vi "Cauchy PDF.vi"(9 "b":dbl=1.0, 10 "a":dbl, 11 "x":dbl) -> (0 "error":i32, 3 "pdf(x)":dbl=0.3183098861837907)   [LabVIEW 2014, in "NI_Gmath.lvlib"]
doc: "Computes the continuous probability density function (PDF) of various distributions. You must manually select the polymorphic instance to use."
uses:
  NI_Gmath.lvlib
  st_error_code.ctl
panel:
  # "Cauchy PDF"
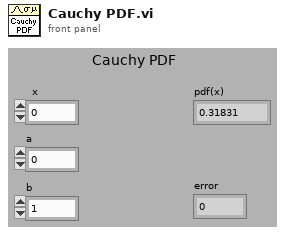
[diagram p1: front panel]
types:
  T1 = typedef "NI_Gmath.lvlib/st_error_code.ctl" = i32
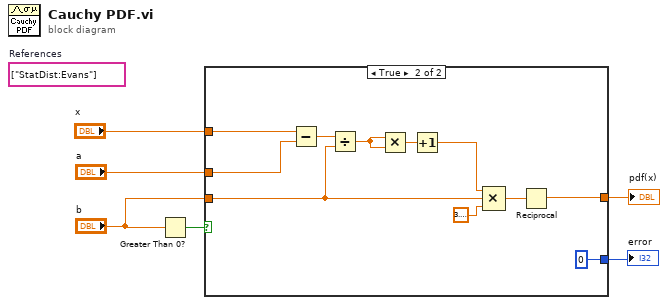
[diagram p0: block diagram]
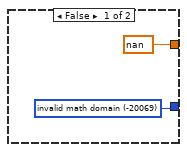
[diagram p2: hidden frame]
diagram:
  (unwired) string[] ["StatDist:Evans"]  # References
  n1 = Greater Than 0?(x="b") -> (x > 0?=w1:bool)
  n2 = case shown="True" w1 {
    tunnel: "b" -> [_ w12]
    tunnel: [w7 0 ("invalid math domain")] -> w6
    tunnel: [nan w9] -> w5
    tunnel: "x" -> [_ w18]
    tunnel: "a" -> [_ w17]
    frame False {
      w7 = T1 -20069 items=["invalid math domain"=-20069, "Fourier interpolation size m >= n"=-20070, "empty array"=-20003] ("stat interp error code")
    }
    frame True {
      n3 = Subtract(x=w18, y=w17) -> (x-y=w16:dbl)
      n4 = Divide(x=w16, y=w12) -> (x/y=w15:dbl)
      n5 = Multiply(x=w15, y=w15) -> (x*y=w14:dbl)
      n6 = Increment(x=w14) -> (x+1=w13:dbl)
      n7 = Compound Arithmetic op=MULTIPLY(w13, w12, 3.141592653589793) -> (w10:dbl)
      n8 = Reciprocal(x=w10) -> (1/x=w9:dbl)
    }
  }
  "pdf(x)" <- w5
  "error" <- w6
